vi "SetField.vi"(9 "Poly Coeffs":dbl[](array[numeric]), 10 "Field Setpoint":dbl, 11 "PS GPIB Address":string="12") -> ()   [LabVIEW 2015]
uses:
  <vilib>/Analysis/polynomials.llb/Scalar Polynomial Evaluation (DBL).vi
  <vilib>/Analysis/NI_AALPro.lvlib
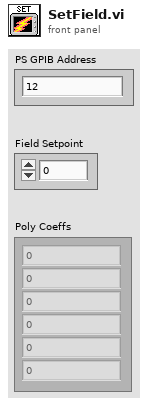
[diagram p1: front panel]
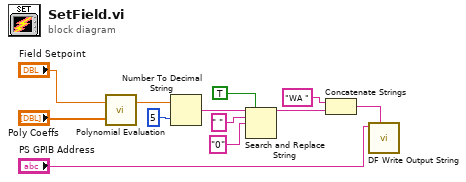
[diagram p0: block diagram]
diagram:
  n1 = call-poly <vilib>:"Polynomial Evaluation.vi"("P(x)"="Poly Coeffs", "a"="Field Setpoint") -> ("P(a)"=w10:dbl)  [unwired: 1 out]
  n2 = Number To Decimal String(number=w10, width (-)=i16 5) -> (decimal integer string=w5:string)
  n3 = Search and Replace String(replace all?=TRUE ("replace all? (F)"), input string=w5, search string=" ", replace string="0" ("replace string (\"\")")) -> (result string=w1:string)  [unwired: 4 in, 3 out]
  n4 = Concatenate Strings("WA " ("string"), w1) -> (w6:string)
  n5 = call "DF Write Output String"("Write String"=w6, "GPIB Address"="PS GPIB Address") -> ()  [unwired: 7 in]
